vi "Config CDMA IQ Mapping.vi"(0 "VISA Resource Name":refnum<visa-resource-name>, 5 "Mapping  (0: Normal)":u16(ring) items=["Normal", "Inverted"], 11 "error in (no error)":errorcluster {"code" format="%.0x"}) -> (4 "VISA Resource Name Out":refnum<visa-resource-name>, 15 "error out":errorcluster {"code" format="%.0x"})   [LabVIEW 2012, in "Agilent ESG Series.lvlib"]
doc: "This VI selects whether the Q output will be normal or inverted.\n\nNotes:\n(1) This VI is supported for Agilent E4438C with option 401 only."
uses:
  <instrlib>/Agilent ESG Series/Agilent ESG Series.lvlib
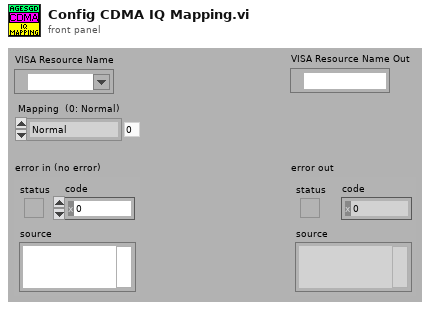
[diagram p1: front panel]
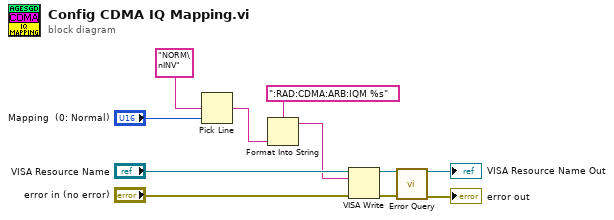
[diagram p0: block diagram]
diagram:
  n1 = Pick Line(multi-line string="NORM\nINV", line index="Mapping  (0: Normal)") -> (output string=w4:string)  [unwired: 1 in]
  n2 = Format Into String(format string=":RAD:CDMA:ARB:IQM %s", w4) -> (resulting string=w1:string)  [unwired: 2 in, 1 out]
  n3 = VISA Write(VISA resource name="VISA Resource Name", write buffer=w1, error in (no error)="error in (no error)") -> (VISA resource name out=w7:refnum<visa-resource-name>, error out=w6:errorcluster)  [unwired: 1 out]
  n4 = call <instrlib>:"Error Query.vi"("VISA Resource Name"=w7, "error in (no error)"=w6) -> ("VISA Resource Name Out"=→"VISA Resource Name Out":refnum<visa-resource-name>, "error out"=→"error out":errorcluster)  [unwired: 10 in, 2 out]
